vi "Read Exception Status.vi"(8 "error in (no error)":errorcluster, 11 "Modbus slave in":refnum<class "Modbus Master CR API.lvclass">) -> (0 "error out":errorcluster, 2 "exception status":u8, 3 "Modbus slave out":refnum<class "Modbus Master CR API.lvclass">)   [LabVIEW 2021, in "Modbus Master CR API.lvclass"]
doc: "Returns the exception status of a Modbus slave. The exception status is a set of eight status bits. Each status bit stands for an exception."
uses:
  Modbus Master CR API.lvclass
  Modbus Master CR API.lvclass/Modbus Master CR API.ctl
  Data Model/Device Data Model.lvclass
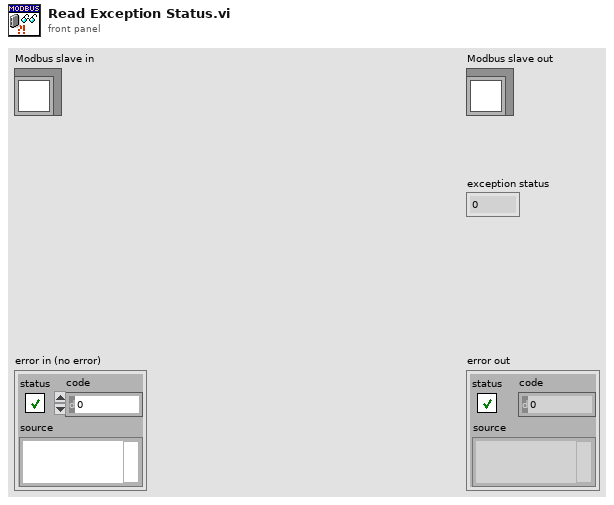
[diagram p1: front panel]
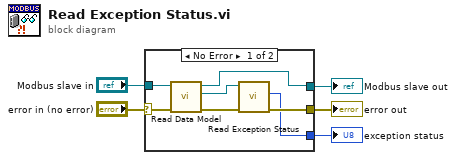
[diagram p0: block diagram]
diagram:
  n1 = case shown="No Error" "error in (no error)" {
    selector: "error in (no error)" -> [w10 w13]
    tunnel: "Modbus slave in" -> [w6 w14]
    tunnel: [w7 w14] -> w4
    tunnel: [w12 w13] -> w3
    tunnel: [w11 _] -> w2
    frame No Error {
      n2 = call "Read Data Model.vi"("error in (no error)"=w10, "Modbus slave in"=w6) -> ("error out"=w9:errorcluster, "device data model"=w8:refnum<class "Device Data Model.lvclass">, "Modbus slave out"=w7:refnum<class "Modbus Master CR API.lvclass">)  [unwired: 7 in]
      n3 = call-dynamic "Read Exception Status.vi"("error in"=w9, "device data model in"=w8) -> ("error out"=w12:errorcluster, "exception status"=w11:u8)  [unwired: 7 in, 1 out]
    }
    frame Error {
    }
  }
  "error out" <- w3
  "Modbus slave out" <- w4
  "exception status" <- w2
